vi "Send Receive.vi"(5 "Time Out (100 ms)":i32=100, 7 "Max Retries  (10)":i32=10, 8 "Error In":errorcluster, 9 "Bytes To Read (0)":u8, 10 "Data":u8[](array[numeric]), 11 "ChipKit Resource":T1={"COM Port"="", "Board Type"=enum."ChipKit Uno32", "Connection Type"=enum."USB / Serial", "Baud Rate (115200)"=15, "Bytes Per Packet (15)"=15}) -> (0 "Error Out":errorcluster, 2 "Read Buffer":string, 3 "ChipKit Resource":T1={"COM Port"="", "Board Type"=enum."ChipKit Uno32", "Connection Type"=enum."USB / Serial", "Baud Rate (115200)"=15, "Bytes Per Packet (15)"=15})   [LabVIEW 2011, in "LabVIEW Interface for ChipKit.lvlib"]
uses:
  LabVIEW Interface for ChipKit.lvlib
  Private/Type Defs/Chipkit Resource.ctl
  Private/Type Defs/Board Type.ctl
  Private/Type Defs/Connection Type.ctl
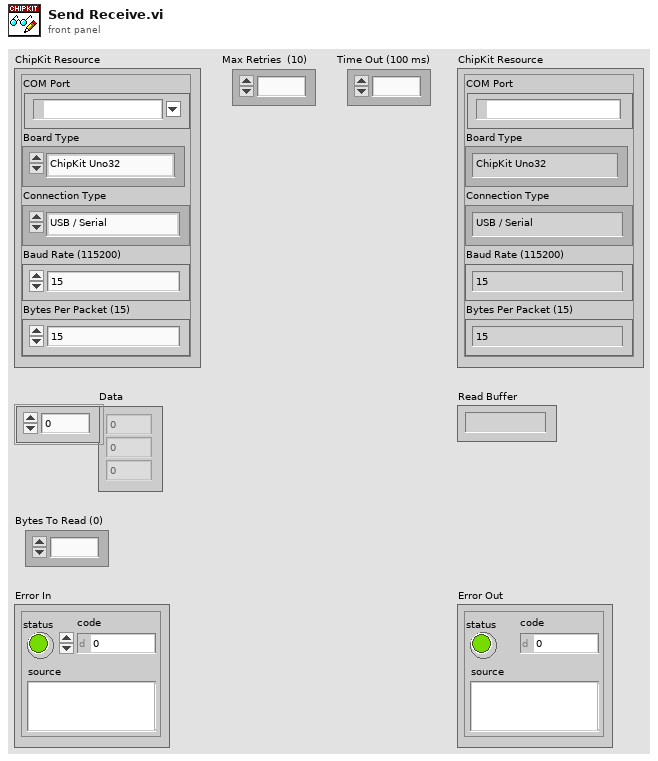
[diagram p1: front panel]
types:
  T1 = typedef "LabVIEW Interface for ChipKit.lvlib/Chipkit Resource.ctl" = cluster{"COM Port":refnum<visa-resource-name>, "Board Type":T2, "Connection Type":T3, "Baud Rate (115200)":u32, "Bytes Per Packet (15)":u32}
  T2 = typedef "LabVIEW Interface for ChipKit.lvlib/Board Type.ctl" = enum16{"ChipKit uC32", "ChipKit Uno32", "ChipKit Max32"}
  T3 = typedef "LabVIEW Interface for ChipKit.lvlib/Connection Type.ctl" = enum8{"USB / Serial", "XBEE", "BlueSmirf (Bluetooth)"}
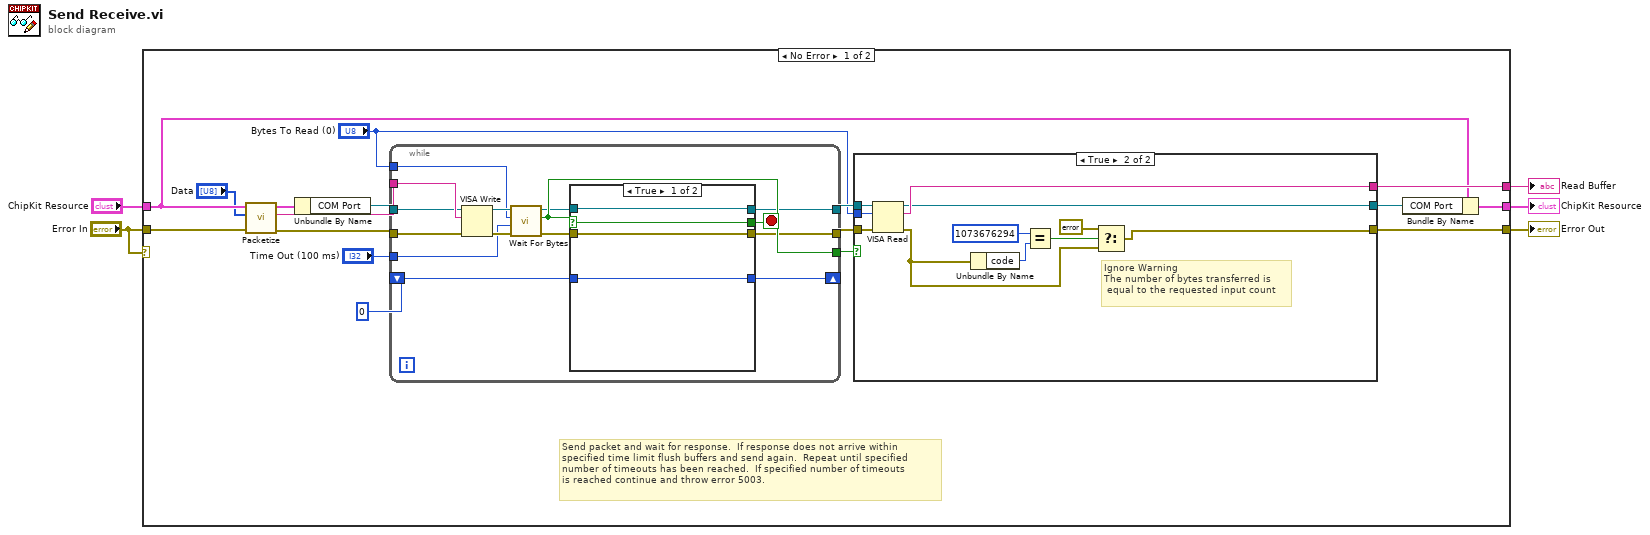
[diagram p0: block diagram]
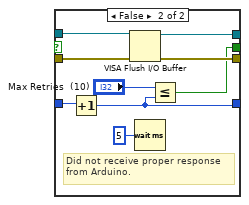
[diagram p2: hidden frame]
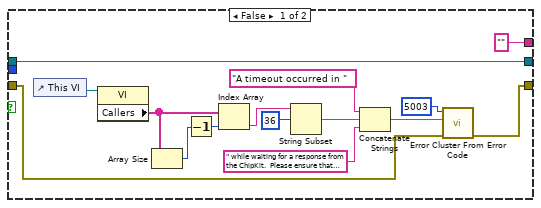
[diagram p3: hidden frame]
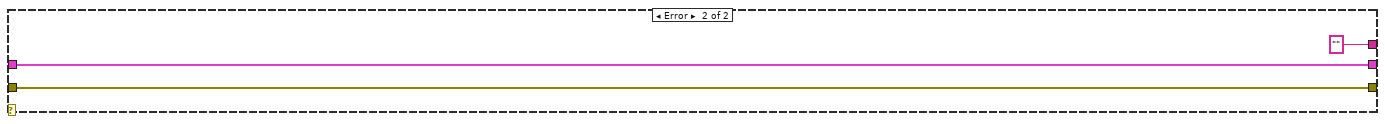
[diagram p4: hidden frame]
diagram:
  n1 = case shown="No Error" "Error In" {
    tunnel: [w22 w78] -> w5
    tunnel: [w20 "" ("read buffer")] -> w4
    tunnel: "Error In" -> [w8 w78]
    tunnel: "ChipKit Resource" -> [w10 w79]
    tunnel: [w16 w79] -> w2
    frame No Error {
      # "Send packet and wait for response.  If response does not arrive within \nspecified time limit flush buffers and send again.  Repeat until specified \nnumber of timeouts has been reached.  If specified number of timeouts\nis reached continue and throw error 5003."
      n2 = call "Packetize.vi"("Error In"=w8, "Data"="Data", "Arduino Resource"=w10) -> ("Error Out"=w9:errorcluster, "Packet"=w21:string, "Arduino Resource"=w11:T1)  [unwired: 6 in]
      n3 = Unbundle By Name(w11) -> ("COM Port"=w18:refnum<visa-resource-name>)
      n4 = while {
        tunnel: w21 -> [w37]
        tunnel: [w25] -> w19
        tunnel: w9 -> [w34]
        tunnel: w18 -> [w33]
        tunnel: "Bytes To Read (0)" -> [w32]
        tunnel: "Time Out (100 ms)" -> [w31]
        tunnel: [w27] -> w13
        shift-right: [w29] -> _
        shift-left: 0 -> [w30]
        tunnel: [w23] -> w6
        stop <- w28 stop-if-true
        n5 = VISA Write(VISA resource name=w33, write buffer=w37, error in (no error)=w34) -> (VISA resource name out=w35:refnum<visa-resource-name>, error out=w36:errorcluster)  [unwired: 1 out]
        n6 = call "Wait For Bytes.vi"("Error In"=w36, "Time Out (100 ms)"=w31, "Bytes To Read"=w32, "VISA resource name"=w35) -> ("Error Out"=w26:errorcluster, "Bytes Available?"=w27:bool, "VISA resource name"=w24:refnum<visa-resource-name>)  [unwired: 5 in]
        n7 = case shown="True" w27 {
          selector: w27 -> [w40 _]
          tunnel: w30 -> [w41 w50]
          tunnel: [w41 w43] -> w29
          tunnel: [w40 w42] -> w28
          tunnel: w26 -> [w38 w48]
          tunnel: [w39 w47] -> w25
          tunnel: w24 -> [w39 w46]
          tunnel: [w38 w45] -> w23
          frame True {
          }
          frame False {
            # "Did not receive proper response\nfrom Arduino."
            n8 = Increment(x=w50) -> (x+1=w43:i32)
            n9 = VISA Flush I/O Buffer(VISA resource name=w46, error in (no error)=w48) -> (VISA resource name out=w47:refnum<visa-resource-name>, error out=w45:errorcluster)  [unwired: 1 in]
            n10 = Wait (ms)(milliseconds to wait=u32 5) -> ()  [unwired: 1 out]
            n11 = Less Or Equal?(x="Max Retries  (10)", y=w43) -> (x <= y?=w42:bool)
          }
        }
      }
      n12 = case shown="True" w13 {
        tunnel: [w55 w66] -> w22
        tunnel: ["" ("read buffer") w76] -> w20
        tunnel: w19 -> [w65 w75]
        tunnel: [w65 w74] -> w17
        tunnel: "Bytes To Read (0)" -> [_ w73]
        tunnel: w6 -> [w54 w72]
        frame False {
          n13 = control-ref of="This VI"() -> (w60:refnum<vi>)
          n14 = property class="VI"(reference=w60) -> ("Callers"=w53:string[])  [unwired: 1 in, 2 out]
          n15 = Array Size(array=w53) -> (size(s)=w51:i32)
          n16 = Decrement(x=w51) -> (x-1=w52:i32)
          n17 = Index Array(array=w53, index=w52) -> (element=w57:string)
          n18 = String Subset(string=w57, offset (0)=36) -> (substring=w56:string)  [unwired: 1 in]
          n19 = Concatenate Strings("A timeout occurred in ", w56, " while waiting for a response from the ChipKit.  Please ensure that the ChipKit is connected to the host computer, has adequate power and that the COM Port, Board Type, and Baud Rate passed to the Init.vi are correct." ("source")) -> (w62:string)
          n20 = call <vilib>:"Error Cluster From Error Code.vi"("error in (no error)"=w54, "error message (\"\")"=w62, "error code (0)"=5003) -> ("error out"=w55:errorcluster)  [unwired: 6 in]
        }
        frame True {
          # "Ignore Warning\nThe number of bytes transferred is\n equal to the requested input count"
          n21 = VISA Read(VISA resource name=w75, byte count=w73, error in (no error)=w72) -> (VISA resource name out=w74:refnum<visa-resource-name>, read buffer=w76:string, error out=w67:errorcluster)  [unwired: 1 out]
          n22 = Unbundle By Name(w67) -> ("code"=w70:i32)
          n23 = Equal?(x=1073676294 ("[error code] (0)"), y=w70) -> (x = y?=w69:bool)
          n24 = Select(t=errorcluster {"status"=FALSE, "code"=0, "source"=""} ("error out"), s=w69, f=w67) -> (s? t:f=w66:errorcluster)
        }
      }
      n25 = Bundle By Name(cluster=w10, "COM Port"=w17) -> (w16:T1)
    }
    frame Error {
    }
  }
  "Error Out" <- w5
  "Read Buffer" <- w4
  "ChipKit Resource" <- w2
